vi "TDD11_22_seperate.vi"(10 "paraLength":dbl, 11 "pairIndex":dbl) -> (3 "is TDD11?":bool)   [LabVIEW 2011]
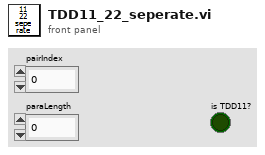
[diagram p1: front panel]
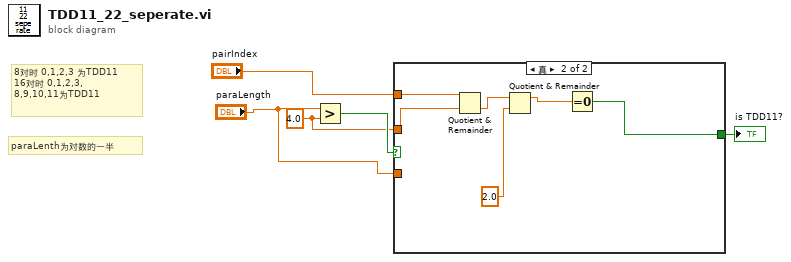
[diagram p0: block diagram]
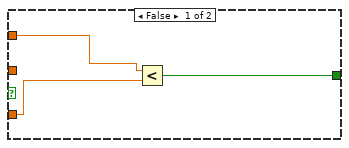
[diagram p2: hidden frame]
diagram:
  w2 = 4.0 ("y")
  # "paraLenth为对数的一半"
  # "8对时 0,1,2,3 为TDD11\n16对时 0,1,2,3,\n8,9,10,11为TDD11"
  n1 = Greater?(x="paraLength", y=w2) -> (0:w5:bool)
  n2 = case shown="真" w5 {
    tunnel: "pairIndex" -> [w8 w14]
    tunnel: "paraLength" -> [w7 _]
    tunnel: [w6 w9] -> w1
    tunnel: w2 -> [_ w13]
    frame False {
      n3 = Less?(x=w8, y=w7) -> (x < y?=w6:bool)
    }
    frame True {
      n4 = Quotient & Remainder(x=w14, y=w13) -> (floor(x/y)=w12:dbl)  [unwired: 1 out]
      n5 = Quotient & Remainder(x=w12, y=2.0) -> (x-y*floor(x/y)=w10:dbl)  [unwired: 1 out]
      n6 = Equal To 0?(x=w10) -> (x = 0?=w9:bool)
    }
  }
  "is TDD11?" <- w1
